vi "Write Paramaters.vi"(8 "error in (no error)":errorcluster, 9 "Parameter Values":T1, 10 "Parameter Indexes":T2, 11 "data table in":T3) -> (0 "error out":errorcluster, 3 "data table out":T3)   [LabVIEW 2015, in "Sequencer Module tests.lvlib"]
uses:
  Sequencer Module tests.lvlib
  <vilib>/NI/Tag Bus/table/data table.ctl
  Parameters Indexes.ctl
  Parameters.ctl
  <vilib>/NI/Tag Bus/table/data polymorphs/write one/write String.vi
  <vilib>/NI/Tag Bus/table/data polymorphs/write one/write Boolean.vi
  <vilib>/NI/Tag Bus/table/data table.lvlib
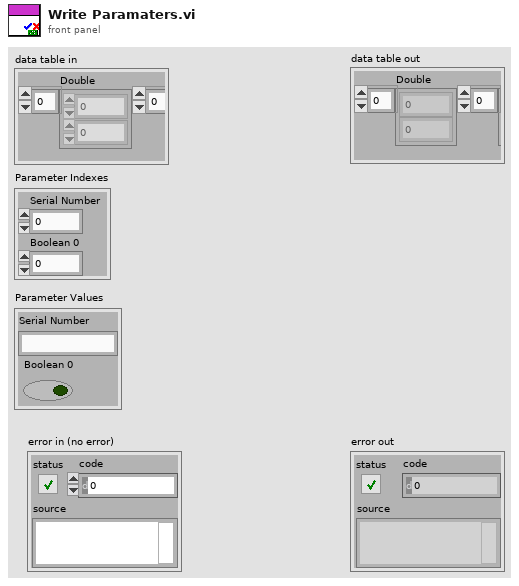
[diagram p1: front panel]
types:
  T1 = typedef "Parameters.ctl" = cluster{"Serial Number":string, "Boolean 0":bool}
  T2 = typedef "Parameters Indexes.ctl" = cluster{"Serial Number":i32, "Boolean 0":i32}
  T3 = typedef "tag bus.lvlib/data table.lvlib/data table.ctl" = cluster{"Double":dbl[], "Single":sgl[], "I64":i64[], "I32":i32[], "I16":i16[], "I8":i8[], "U64":u64[], "U32":u32[], "U16":u16[], "U8":u8[], "Boolean":bool[], "String":string[], "Array of Double":cluster{"DBL Array":dbl[]}[], "Array of Single":cluster{"SGL Array":sgl[]}[], "Array of I64":cluster{"I64 Array":i64[]}[], "Array of I32":cluster{"I32 Array":i32[]}[], "Array of I16":cluster{"I16 Array":i16[]}[], "Array of I8":cluster{"I8 Array":i8[]}[], "Array of U64":cluster{"U64 Array":u64[]}[], "Array of U32":cluster{"U32 Array":u32[]}[], "Array of U16":cluster{"U16 Array":u16[]}[], "Array of U8":cluster{"U8 Array":u8[]}[], "Array of Boolean":cluster{"Boolean Array":bool[]}[], "Array of String":cluster{"String Array":string[]}[]}
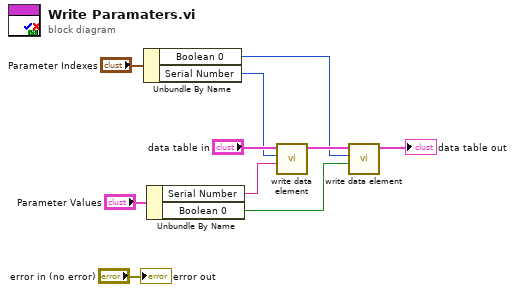
[diagram p0: block diagram]
diagram:
  n1 = Unbundle By Name("Parameter Indexes") -> ("Boolean 0"=w3:i32, "Serial Number"=w4:i32)
  n2 = Unbundle By Name("Parameter Values") -> ("Serial Number"=w5:string, "Boolean 0"=w1:bool)
  n3 = call-poly <vilib>:"write data element.vi"("value"=w5, "index"=w4, "data table in"="data table in") -> ("data table out"=w8:T3)  [unwired: 8 in]
  n4 = call-poly <vilib>:"write data element.vi"("value"=w1, "index"=w3, "data table in"=w8) -> ("data table out"=→"data table out":T3)  [unwired: 8 in]
  "error out" <- "error in (no error)"
